vi "Query.vi"(8 "error in":errorcluster, 10 "Query":string, 11 "DB-ADO in":refnum<class "DB-ADO.lvclass">) -> (0 "error out":errorcluster, 1 "Packed Metadata":variant, 2 "Return Data":string[][](array[string]), 3 "DB-ADO out":refnum<class "DB-ADO.lvclass">, 4 "Field Names":string[](array[string]))   [LabVIEW 2022 SP3, in "hse-db-ado.lvlib" / "DB-ADO.lvclass"]
doc: "Send a SQL-query and return the answer. Return data is a 2D-array of strings wraped in variants.\n\n____\nHAMPEL SOFTWARE ENGINEERING v1.4.0 (2023-12-19 09:52)"
uses:
  DB-ADO.lvclass
  DB-ADO.lvclass/DB-ADO.ctl
  ADO-DB-Drivers/ADO-DB-Driver.lvlib
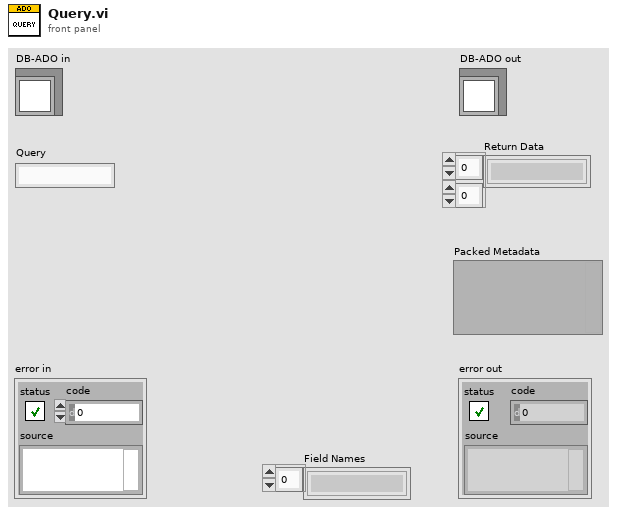
[diagram p1: front panel]
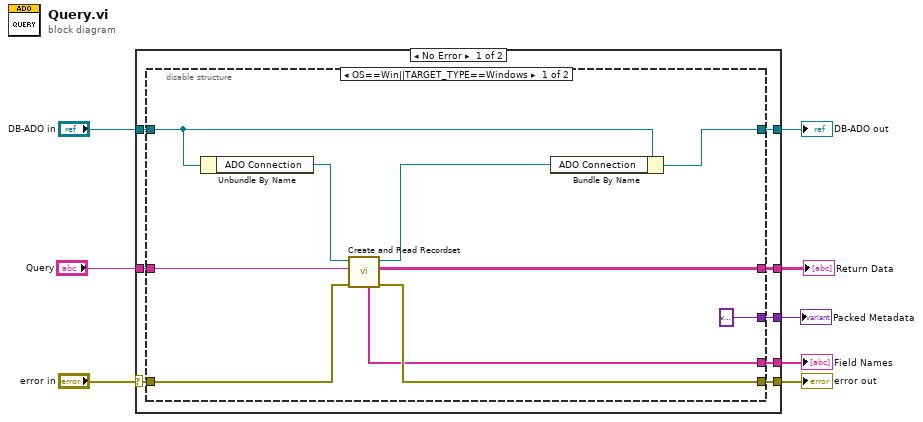
[diagram p0: block diagram]
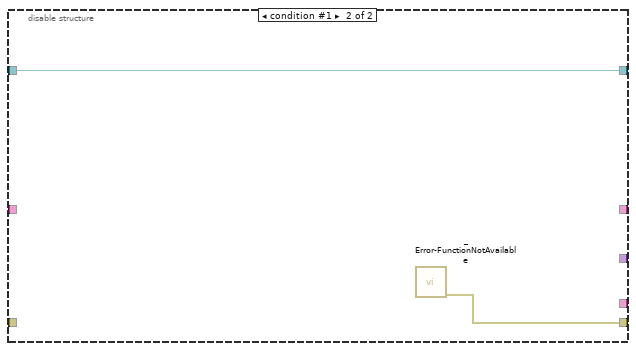
[diagram p2: hidden frame]
diagram:
  n1 = case shown="No Error" "error in" {
    selector: "error in" -> [w16 w30]
    tunnel: [w15 w30] -> w7
    tunnel: [w12 w29] -> w5
    tunnel: "DB-ADO in" -> [w13 w29]
    tunnel: "Query" -> [w14 _]
    tunnel: [w11 _] -> w2
    tunnel: [w10 _] -> w3
    tunnel: [w9 _] -> w1
    frame No Error {
      n2 = disable-structure shown="OS==Win||TARGET_TYPE==Windows" {
        disable-tunnel: w16 -> [w26 _]
        disable-tunnel: [w25 w27] -> w15
        disable-tunnel: w14 -> [w23 _]
        disable-tunnel: w13 -> [w22 w28]
        disable-tunnel: [w21 w28] -> w12
        disable-tunnel: [w18 _] -> w11
        disable-tunnel: [w19 _] -> w10
        disable-tunnel: [variant _] -> w9
        frame condition #0 (active) {
          n3 = Unbundle By Name(w22) -> ("ADO Connection"=w24:refnum<k7>)
          n4 = call "Create and Read Recordset.vi"("error in (no error)"=w26, "Source"=w23, "Connection In"=w24) -> ("error out"=w25:errorcluster, "Selection Data"=w18:string[][], "Connection Out"=w20:refnum<k7>, "Field Names Fetched"=w19:string[])  [unwired: 4 in, 1 out]
          n5 = Bundle By Name(cluster=w22, "ADO Connection"=w20) -> (w21:refnum<class "DB-ADO.lvclass">)
        }
        frame condition #1 {
          n6 = call "_Error-FunctionNotAvailable.vi"() -> ("error out"=w27:errorcluster)  [unwired: 11 in]
        }
      }
    }
    frame Error {
    }
  }
  "error out" <- w7
  "DB-ADO out" <- w5
  "Field Names" <- w3
  "Return Data" <- w2
  "Packed Metadata" <- w1
